vi "EMSG_SelectRef_ByName.vi"(8 "Error in":errorcluster caption="Error in (no error)", 9 "Name":string, 10 "NameHistory":string[](array[string]), 11 "MsgEventHistory":refnum<user-event>[](array[refnum])) -> (0 "Error out":errorcluster, 3 "User Event out":refnum<user-event>)   [LabVIEW 2014, in "EventMsg.lvclass"]
uses:
  EventMsg.lvclass
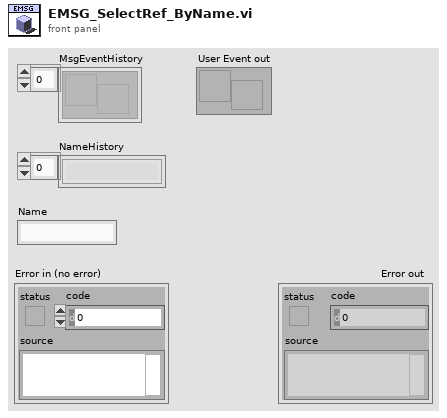
[diagram p1: front panel]
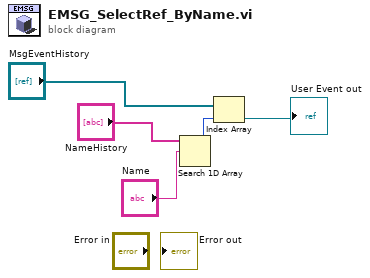
[diagram p0: block diagram]
diagram:
  n1 = Search 1D Array(1D array="NameHistory", element="Name") -> (index of element=w5:i32)  [unwired: 1 in]
  n2 = Index Array(array="MsgEventHistory", index=w5) -> (element=→"User Event out":refnum<user-event>)
